vi "Initialize AO.vi"(0 "DAQ":refnum<class "DAQ.lvclass">, 1 "N Ch 1 task":bool=TRUE, 5 "DAQNode Dict":T1, 7 "AO Channels":T2[](array[typedef]) {"Conversion"."ScaleOffset" format="%.3f"; "Conversion"."MinEngUnit" format="%.3f"; "Conversion"."MaxEngUnit" format="%.3f"; "Conversion"."MinSignal" format="%.3f"; "Conversion"."MaxSignal" format="%.3f"}, 11 "error in":errorcluster, 14 "Simulate":bool) -> (4 "DAQ out":refnum<class "DAQ.lvclass">, 6 "DAQNode Dict out":T1, 15 "error out":errorcluster)   [LabVIEW 2022 SP3, in "DAQ.lvclass"]
doc: "Developed by Kevin Thompson\nkevin@thompsonengineering.net\n\nCopyright 2015\nThompson Engineering, LLC"
uses:
  DAQ.lvclass
  DataTypes/TD AO Channel--cluster.ctl
  DataTypes/TD DataValueConversion--cluster.ctl
  <vilib>/TELLC/Dynamic CVT API/TD Dynamic CVT DVR--ref.ctl
  DAQ.lvclass/DAQ.ctl
  Accessors/Set AO SchemNames.vi
  Accessors/Set AO IONames.vi
  <vilib>/Utility/error.llb/Trim Whitespace One-Sided.vi
  <vilib>/DAQmx/create/channels.llb/DAQmx Create Channel (AO-Voltage-Basic).vi
panel:
  out "names out":string
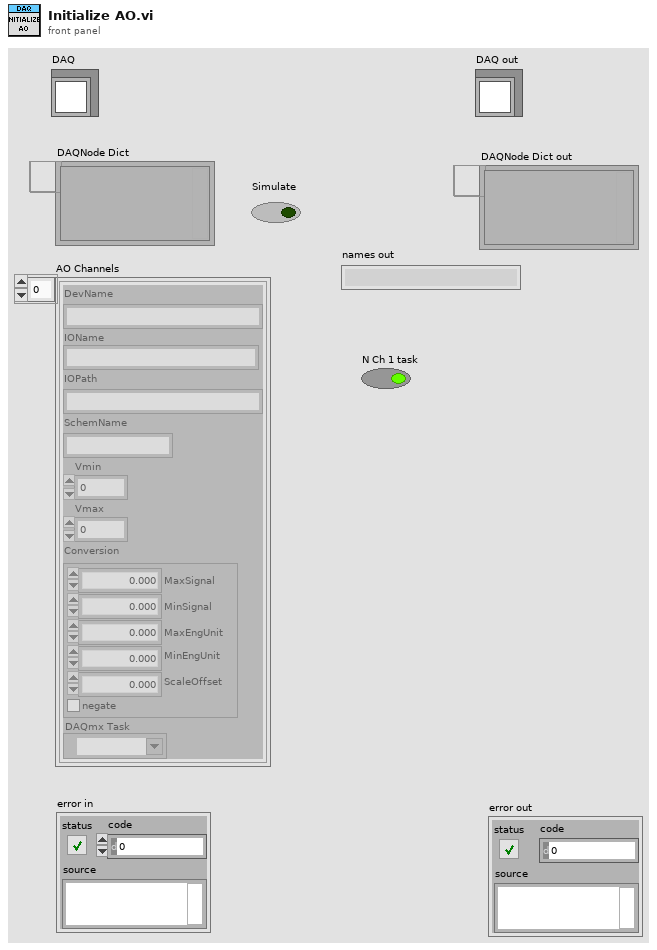
[diagram p1: front panel]
types:
  T1 = typedef "TD Dynamic CVT DVR--ref.ctl" = refnum<data-value>
  T2 = typedef "DAQ.lvclass/TD AO Channel--cluster.ctl" = cluster{"DevName":string, "IOName":string, "IOPath":string, "SchemName":string, "Vmin":dbl, "Vmax":dbl, "Conversion":T3, "DAQmx Task":refnum<k21>}
  T3 = typedef "DAQ.lvclass/TD DataValueConversion--cluster.ctl" = cluster{"MaxSignal":dbl, "MinSignal":dbl, "MaxEngUnit":dbl, "MinEngUnit":dbl, "ScaleOffset":dbl, "negate":bool}
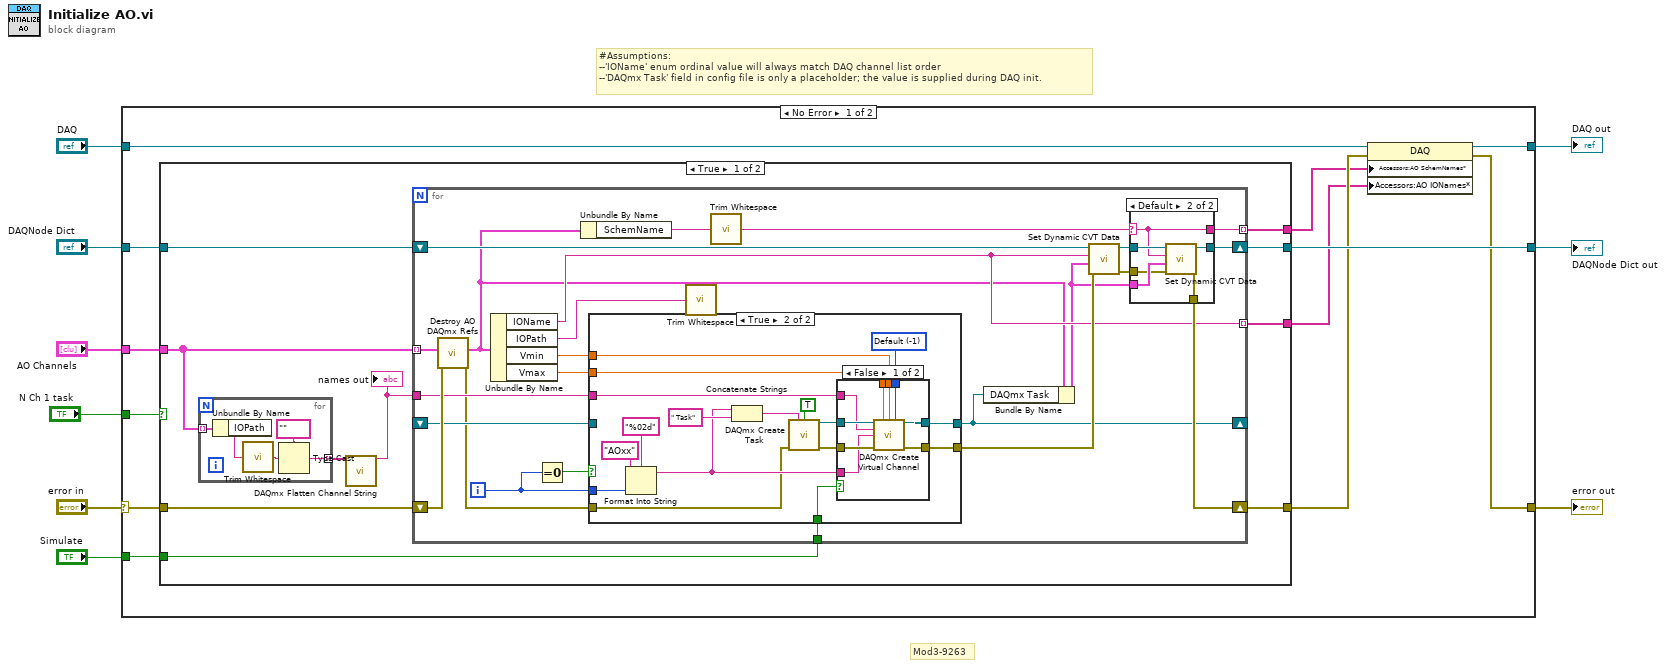
[diagram p0: block diagram]
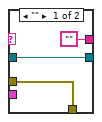
[diagram p4: hidden frame]
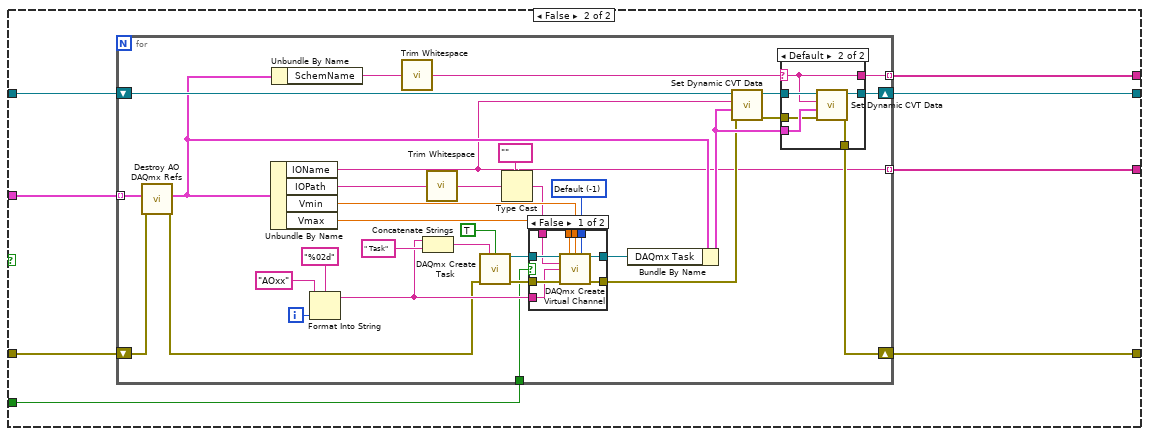
[diagram p5: hidden frame]
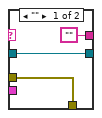
[diagram p6: hidden frame]
diagram:
  # "Mod3-9263"
  # "#Assumptions:\n--'IOName' enum ordinal value will always match DAQ channel list order\n--'DAQmx Task' field in config file is only a placeholder; the value is supplied during DAQ init."
  n1 = case shown="No Error" "error in" {
    selector: "error in" -> [w20 w163]
    tunnel: "AO Channels" -> [w18 _]
    tunnel: "DAQNode Dict" -> [w21 w162]
    tunnel: [w13 w163] -> w8
    tunnel: [w19 w162] -> w7
    tunnel: "Simulate" -> [w17 _]
    tunnel: "DAQ" -> [w15 w161]
    tunnel: [w14 w161] -> w3
    tunnel: "N Ch 1 task" -> [w16 _]
    frame No Error {
      n2 = case shown="True" w16 {
        tunnel: w21 -> [w31 w107]
        tunnel: w20 -> [w30 w106]
        tunnel: [w29 w105] -> w19
        tunnel: w18 -> [w27 w104]
        tunnel: [w28 w103] -> w12
        tunnel: w17 -> [w25 w102]
        tunnel: [w23 w101] -> w11
        tunnel: [w22 w100] -> w10
        frame True {
          n3 = for {
            tunnel: w27 -> [w36] mode=indexing
            tunnel: [w32] -> w24 mode=indexing
            n4 = Unbundle By Name(w36) -> ("IOPath"=w33:string)
            n5 = call <vilib>:"Trim Whitespace.vi"("string"=w33) -> ("trimmed string"=w34:string)  [unwired: 1 in]
            n6 = Type Cast(type=tag "" ("physical channels"), x=w34) -> (*(type *) &x=w32:tag)
          }
          n7 = call <vilib>:"DAQmx Flatten Channel String.vi"("names in"=w24) -> ("names out"=w26:string)  [unwired: 13 in, 1 out]
          "names out" <- w26
          n8 = for {
            tunnel: w27 -> [w56] mode=indexing
            shift-right: [w49] -> w28
            shift-left: w30 -> [w55]
            shift-right: [w52] -> w29
            shift-left: w31 -> [w57]
            tunnel: w25 -> [w54]
            tunnel: [w46] -> w23 mode=indexing
            tunnel: [w45] -> w22 mode=indexing
            tunnel: w26 -> [w42]
            shift-right: [w39] -> _
            shift-left: _ -> [w38]
            i -> [w40]
            n9 = call "Destroy AO DAQmx Refs.vi"("error in (no error)"=w55, "AO"=w56) -> ("error out"=w37:errorcluster, "AO OUT"=w44:T2)  [unwired: 8 in]
            n10 = Unbundle By Name(w44) -> ("IOName"=w45:string, "IOPath"=w58:string, "Vmin"=w59:dbl, "Vmax"=w60:dbl)
            n11 = Equal To 0?(x=w40) -> (x = 0?=w41:bool)
            n12 = Unbundle By Name(w44) -> ("SchemName"=w51:string)
            n13 = case shown="True" w41 {
              tunnel: w60 -> [_ w79]
              tunnel: w59 -> [_ w78]
              tunnel: w40 -> [_ w76]
              tunnel: [w62 w73] -> w39
              tunnel: w54 -> [_ w68]
              tunnel: [w61 w65] -> w48
              tunnel: w42 -> [_ w63]
              tunnel: w38 -> [w62 _]
              tunnel: w37 -> [w61 w64]
              frame False {
              }
              frame True {
                w72 = -1 items=["Default"=-1, "RSE"=10083, "Differential"=10106, "Pseudodifferential"=12529] ("output terminal configuration")
                n14 = Format Into String(format string="%02d", initial string="AOxx", w76) -> (resulting string=w70:string)  [unwired: 1 in, 1 out]
                n15 = Concatenate Strings(w70, " Task" ("string")) -> (w69:string)
                n16 = call <vilib>:"DAQmx Create Task.vi"("new task name"=w69, "auto cleanup"=TRUE, "error in"=w64) -> ("task out"=w77:refnum<k21>, "error out"=w74:errorcluster)  [unwired: 11 in]
                n17 = case shown="False" w68 {
                  tunnel: w79 -> [w88 _]
                  tunnel: w78 -> [w87 _]
                  tunnel: w77 -> [w86 w90]
                  tunnel: w74 -> [w85 w89]
                  tunnel: [w84 w90] -> w73
                  tunnel: [w83 w89] -> w65
                  tunnel: w72 -> [w82 _]
                  tunnel: w70 -> [w81 _]
                  tunnel: w63 -> [w80 _]
                  frame False {
                    n18 = call-poly <vilib>:"DAQmx Create Virtual Channel.vi"("task in"=w86, "maximum value"=w88, "minimum value"=w87, "output terminal configuration"=w82, "physical channels"=w80, "name to assign"=w81, "error in"=w85) -> ("task out"=w84:refnum<k21>, "error out"=w83:errorcluster)  [unwired: 7 in]
                  }
                  frame True {
                  }
                }
              }
            }
            n19 = call <vilib>:"Trim Whitespace.vi"("string"=w58) -> ()  [unwired: 1 in, 1 out]
            n20 = call <vilib>:"Trim Whitespace.vi"("string"=w51) -> ("trimmed string"=w47:string)  [unwired: 1 in]
            n21 = Bundle By Name(cluster=w44, "DAQmx Task"=w39) -> (w43:T2)
            n22 = call <vilib>:"Set Dynamic CVT Data.vi"("error in (no error)"=w48, "value"=w43, "DataName"=w45, "dCVT DVR"=w57) -> ("error out"=w50:errorcluster, "dCVT DVR out"=w53:T1)  [unwired: 5 in, 1 out]
            n23 = case shown="Default" w47 {
              selector: w47 -> [_ w94]
              tunnel: w53 -> [w93 w99]
              tunnel: [w93 w98] -> w52
              tunnel: w43 -> [_ w97]
              tunnel: w50 -> [w92 w96]
              tunnel: [w92 w95] -> w49
              tunnel: ["" w94] -> w46
              frame "" {
              }
              frame Default {
                n24 = call <vilib>:"Set Dynamic CVT Data.vi"("error in (no error)"=w96, "value"=w97, "DataName"=w94, "dCVT DVR"=w99) -> ("error out"=w95:errorcluster, "dCVT DVR out"=w98:T1)  [unwired: 5 in, 1 out]
              }
            }
          }
        }
        frame False {
          n25 = for {
            tunnel: w104 -> [w124] mode=indexing
            shift-right: [w112] -> w103
            shift-left: w106 -> [w123]
            shift-right: [w117] -> w105
            shift-left: w107 -> [w132]
            tunnel: w102 -> [w121]
            tunnel: [w109] -> w101 mode=indexing
            tunnel: [w108] -> w100 mode=indexing
            i -> [w135]
            w130 = -1 items=["Default"=-1, "RSE"=10083, "Differential"=10106, "Pseudodifferential"=12529] ("output terminal configuration")
            n26 = call "Destroy AO DAQmx Refs.vi"("error in (no error)"=w123, "AO"=w124) -> ("error out"=w122:errorcluster, "AO OUT"=w115:T2)  [unwired: 8 in]
            n27 = Unbundle By Name(w115) -> ("IOName"=w108:string, "IOPath"=w137:string, "Vmin"=w139:dbl, "Vmax"=w140:dbl)
            n28 = Unbundle By Name(w115) -> ("SchemName"=w114:string)
            n29 = Format Into String(format string="%02d", initial string="AOxx", w135) -> (resulting string=w126:string)  [unwired: 1 in, 1 out]
            n30 = call <vilib>:"Trim Whitespace.vi"("string"=w114) -> ("trimmed string"=w110:string)  [unwired: 1 in]
            n31 = Concatenate Strings(w126, " Task" ("string")) -> (w125:string)
            n32 = call <vilib>:"Trim Whitespace.vi"("string"=w137) -> ("trimmed string"=w136:string)  [unwired: 1 in]
            n33 = call <vilib>:"DAQmx Create Task.vi"("new task name"=w125, "auto cleanup"=TRUE, "error in"=w122) -> ("task out"=w138:refnum<k21>, "error out"=w133:errorcluster)  [unwired: 11 in]
            n34 = Type Cast(type=tag "" ("physical channels"), x=w136) -> (*(type *) &x=w128:tag)
            n35 = case shown="False" w121 {
              tunnel: w140 -> [w158 _]
              tunnel: w139 -> [w157 _]
              tunnel: w138 -> [w156 w160]
              tunnel: w133 -> [w155 w159]
              tunnel: [w154 w160] -> w131
              tunnel: [w153 w159] -> w111
              tunnel: w130 -> [w152 _]
              tunnel: w128 -> [w151 _]
              tunnel: w126 -> [w150 _]
              frame False {
                n36 = call-poly <vilib>:"DAQmx Create Virtual Channel.vi"("task in"=w156, "maximum value"=w158, "minimum value"=w157, "output terminal configuration"=w152, "physical channels"=w151, "name to assign"=w150, "error in"=w155) -> ("task out"=w154:refnum<k21>, "error out"=w153:errorcluster)  [unwired: 7 in]
              }
              frame True {
              }
            }
            n37 = Bundle By Name(cluster=w115, "DAQmx Task"=w131) -> (w116:T2)
            n38 = call <vilib>:"Set Dynamic CVT Data.vi"("error in (no error)"=w111, "value"=w116, "DataName"=w108, "dCVT DVR"=w132) -> ("error out"=w113:errorcluster, "dCVT DVR out"=w118:T1)  [unwired: 5 in, 1 out]
            n39 = case shown="Default" w110 {
              selector: w110 -> [_ w144]
              tunnel: w118 -> [w143 w149]
              tunnel: [w143 w148] -> w117
              tunnel: w116 -> [_ w147]
              tunnel: w113 -> [w142 w146]
              tunnel: [w142 w145] -> w112
              tunnel: ["" w144] -> w109
              frame "" {
              }
              frame Default {
                n40 = call <vilib>:"Set Dynamic CVT Data.vi"("error in (no error)"=w146, "value"=w147, "DataName"=w144, "dCVT DVR"=w149) -> ("error out"=w145:errorcluster, "dCVT DVR out"=w148:T1)  [unwired: 5 in, 1 out]
              }
            }
          }
        }
      }
      n41 = property class="DAQ"(reference=w15, error in=w12, "Accessors:AO SchemNames*"=w11, "Accessors:AO IONames*"=w10) -> (reference out=w14:refnum<class "DAQ.lvclass">, error out=w13:errorcluster)
    }
    frame Error {
    }
  }
  "error out" <- w8
  "DAQNode Dict out" <- w7
  "DAQ out" <- w3
